vi "Zthreshholdtesting.vi"() -> ()   [LabVIEW 2019]
uses:
  <userlib>/HapticSTM/HapticSTM.lvlib
panel:
  out "Zthresh":dbl
  in  "stop":bool
  out "current":dbl
  in  "z pos pen":dbl(slide) scale=-100.0..100.0
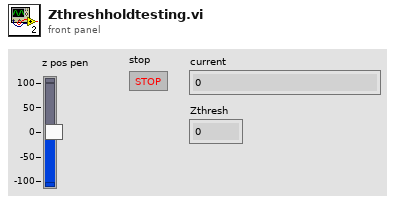
[diagram p1: front panel]
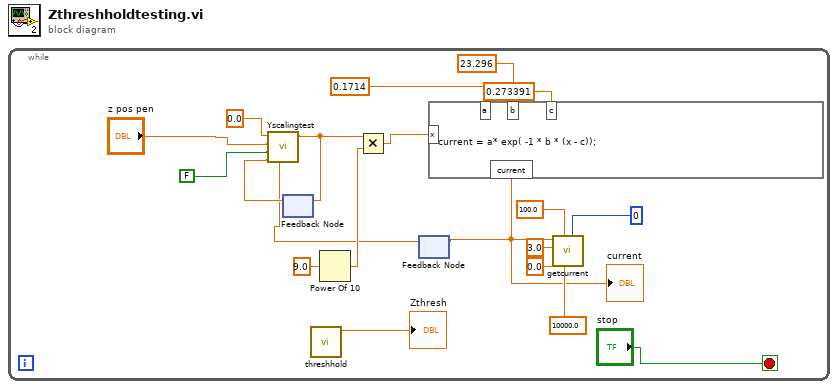
[diagram p0: block diagram]
diagram:
  n1 = while {
    stop <- "stop" stop-if-true
    n2 = feedback #1() -> (w4:dbl)  [unwired: 1 in]
    n3 = call <userlib>:"threshhold.vi"() -> ("function return"=→"Zthresh":dbl)  [unwired: 11 in]
    n4 = Power Of 10(x=9.0) -> (10^x=w10:dbl)
    n5 = feedback #2() -> (w1:dbl)  [unwired: 1 in]
    n6 = call <userlib>:"Yscalingtest.vi"("current"=w1, "Nano Z Read"=w4, "Current Maxed?"=FALSE, "Y"="z pos pen", "Plane Height"=0.0) -> ("y scaled"=w3:dbl)  [unwired: 5 in, 1 out]
    n7 = feedback-in #1(w3) -> ()
    n8 = Multiply(x=w3, y=w10) -> (x*y=w11:dbl)
    n9 = formula code="current = a* exp( -1 * b * (x - c));"("x"=w11, "a"=0.1714 ("input variable"), "b"=23.296 ("input variable"), "c"=0.273391 ("input variable")) -> ("current"=w2:dbl)
    "current" <- w2
    n10 = feedback-in #2(w2) -> ()
    n11 = call <userlib>:"getcurrent.vi"("forcemode"=0, "maxcurrentin"=10000.0, "setpoint"=100.0, "minforcey"=0.0, "maxforcey"=3.0, "currentin"=w2) -> ()  [unwired: 6 in]
  }
